vi "Morphology (Black Hat).vi"(5 "Iterations (Default: 1)":u16=1, 7 "Anchor Point (Default -1,-1 Use Centre)":T2={"x"=-1, "y"=-1}, 8 "error in (no error)":errorcluster, 10 "Structuring Element":bool[][](array[boolean]), 11 "Greyscale Image-Source in":T1) -> (0 "error out":errorcluster, 3 "Greyscale Image-Source":T1)   [LabVIEW 2020, in "image.lvlib"]
doc: "Apply the specified Structuring Element to the Source Image.\n\nUse \"Get Morphology Structuring Element.vi\" to generate common structuring element types."
uses:
  image.lvlib
  common/Image Point (Integer).ctl
  Greyscale Image.ctl
  MorphologyTypes.ctl
  <vilib>/Utility/error.llb/Error Cluster From Error Code.vi
  common/common.lvlib
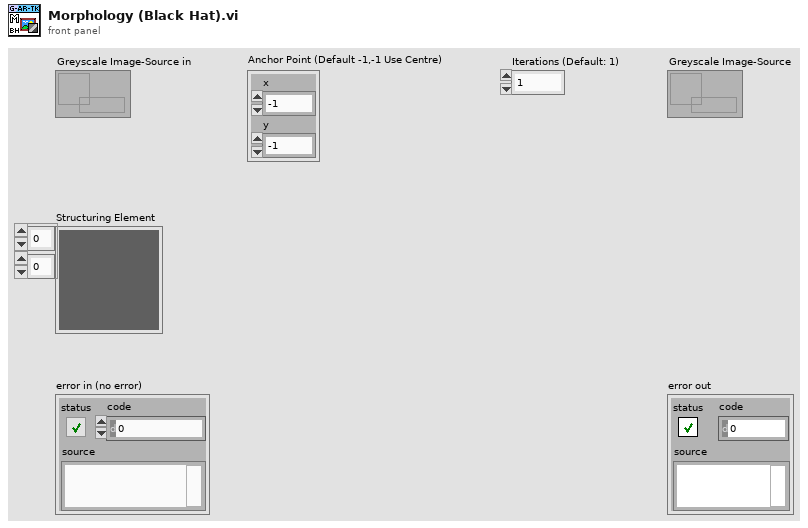
[diagram p1: front panel]
types:
  T1 = typedef "image.lvlib/Greyscale Image.ctl" = refnum<data-value>
  T2 = typedef "common.lvlib/Image Point (Integer).ctl" = cluster{"x":i32, "y":i32}
  T3 = typedef "image.lvlib/MorphologyTypes.ctl" = enum16{"MORPH_ERODE", "MORPH_DILATE", "MORPH_OPEN", "MORPH_CLOSE", "MORPH_GRADIENT", "MORPH_TOPHAT", "MORPH_BLACKHAT", "MORPH_HITMISS"}
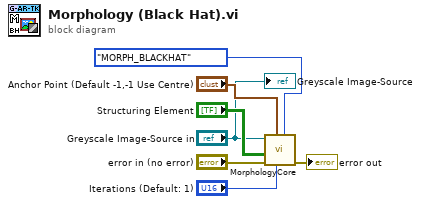
[diagram p0: block diagram]
diagram:
  n1 = call "MorphologyCore.vi"("MorphologyType"=MorphologyTypes."MORPH_BLACKHAT", "Iterations"="Iterations (Default: 1)", "Anchor Point"="Anchor Point (Default -1,-1 Use Centre)", "error in (no error)"="error in (no error)", "Structuring Element"="Structuring Element", "Greyscale Image-Source"="Greyscale Image-Source in") -> ("error out"=→"error out":errorcluster)  [unwired: 5 in]
  "Greyscale Image-Source" <- "Greyscale Image-Source in"
